vi "Post-Install Custom Action.vi"(10 "Variant":variant) -> (0 "error out":errorcluster)   [LabVIEW 2019]
uses:
  <vilib>/Utility/traverseref.llb/TRef TravTarget.ctl
  <vilib>/Utility/traverseref.llb/VI Scripting - Traverse.lvlib
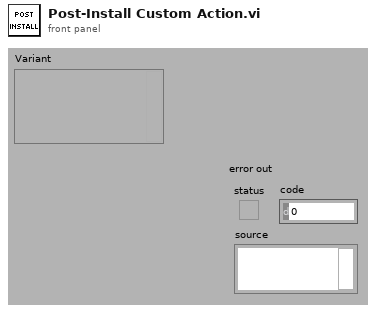
[diagram p1: front panel]
types:
  T1 = typedef "TRef TravTarget.ctl" = enum16{"FP", "BD", "Other"}
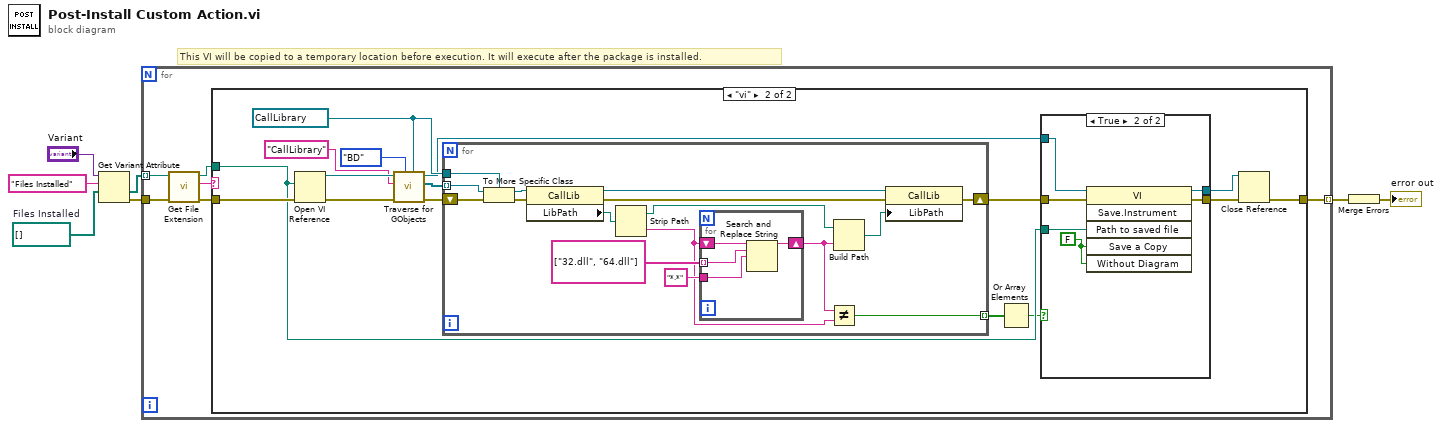
[diagram p0: block diagram]
diagram:
  w5 = path[] []  # Files Installed
  # "This VI will be copied to a temporary location before execution. It will execute after the package is installed."
  n1 = Get Variant Attribute(Variant="Variant", name="Files Installed", default value (empty Variant)=w5) -> (value=w4:path[], error out=w3:errorcluster)  [unwired: 1 in, 2 out]
  n2 = for {
    tunnel: w4 -> [w13] mode=indexing
    tunnel: w3 -> [w9]
    tunnel: [w8] -> w2 mode=indexing
    n3 = call <vilib>:"Get File Extension.vi"("error in (no error)"=w9, "file"=w13) -> ("error out"=w10:errorcluster, "lowercase file extension"=w12:string, "dup file"=w11:path)  [unwired: 5 in, 2 out]
    n4 = case shown="\"vi\"" w12 {
      tunnel: w11 -> [_ w19]
      tunnel: w10 -> [_ w26]
      tunnel: [_ w15] -> w8
      frame "False", Default {
      }
      frame "vi" {
        w22 = refnum<vi> refnum ("Other Refnum")
        n5 = Open VI Reference(vi path=w19, error in (no error)=w26) -> (vi reference=w29:refnum<vi>, error out=w27:errorcluster)  [unwired: 4 in]
        n6 = call <vilib>:"Traverse for GObjects.vi"("Other Refnum"=w22, "Traverse Target"=TRef_TravTarget."BD", "error in (no error)"=w27, "Class Name"="CallLibrary", "VI Refnum"=w29) -> ("error out"=w23:errorcluster, "References"=w24:refnum<vi>[], "dup VI Refnum"=w20:refnum<vi>)  [unwired: 3 in, 1 out]
        n7 = for {
          tunnel: w24 -> [w53] mode=indexing
          tunnel: w22 -> [w51]
          shift-right: [w41] -> w21
          shift-left: w23 -> [w52]
          tunnel: [w38] -> w17 mode=indexing
          n8 = To More Specific Class(target class=w51, reference=w53, error in=w52) -> (specific class reference=w50:refnum<vi>, error out=w49:errorcluster)
          n9 = property class="CallLib"(reference=w50, error in=w49) -> (reference out=w44:refnum<vi>, error out=w43:errorcluster, "LibPath"=w48:path)
          n10 = Strip Path(path=w48) -> (stripped path=w45:path, name=w39:string)
          n11 = for {
            tunnel: string[] ["32.dll", "64.dll"] ("search string") -> [w56] mode=indexing
            tunnel: "*.*" ("search string") -> [w55]
            shift-right: [w54] -> w40
            shift-left: w39 -> [w57]
            n12 = Search and Replace String(input string=w57, search string=w56, replace string=w55) -> (result string=w54:string)  [unwired: 5 in, 3 out]
          }
          n13 = Not Equal?(x=w40, y=w39) -> (x != y?=w38:bool)
          n14 = Build Path(base path=w45, name or relative path=w40) -> (appended path=w42:path)
          n15 = property class="CallLib"(reference=w44, error in=w43, "LibPath"=w42) -> (error out=w41:errorcluster)  [unwired: 1 out]
        }
        n16 = Or Array Elements(Boolean array=w17) -> (logical OR=w16:bool)
        n17 = case shown="True" w16 {
          tunnel: w21 -> [w31 w37]
          tunnel: w20 -> [w30 w36]
          tunnel: w19 -> [_ w35]
          tunnel: [w31 w34] -> w18
          tunnel: [w30 w32] -> w14
          frame False {
          }
          frame True {
            w33 = FALSE ("Save a Copy")
            n18 = invoke class="VI" method="Save.Instrument"(reference=w36, error in=w37, "Path to saved file"=w35, "Save a Copy"=w33, "Without Diagram"=w33) -> (reference out=w32:refnum<vi>, error out=w34:errorcluster)  [unwired: 1 in, 4 out]
          }
        }
        n19 = Close Reference(reference=w14, error in (no error)=w18) -> (error out=w15:errorcluster)
      }
    }
  }
  n20 = Merge Errors(w2) -> (→"error out":errorcluster)
